vi "SendPPMSCommand_Rotator.vi"() -> ()   [LabVIEW 2016]
uses:
  Instance           1 31Saved   SendPPMSCommand_Rotator .vi
panel:
  out "Position while moving":dbl
  in  "Timeout":dbl
  in  "Delay":dbl=5.0
  out "error out":errorcluster
  in  "Slow down code\ndefault = 0":T1(ring)
  in  "Mode":u16(ring) items=["Move to position", "Move to limit", "Redefine current position", ""]
  in  "Position (deg)":dbl
  out "SendPPMSCommand Error 2":i32
  out "PpmsReply 2":string="0.000000"
  in  "PpmsCommand 2":string="$GETONE? 3"
  out "SendPPMSCommand Error":i32=1
  out "PpmsReply":string
  in  "Remote":bool
  in  "IP Address":string="127.0.0.0"
  # "Set Position"
  # "Final Position"
  # "Instrument Connection"
  # "Wait for Position"
  # "Note: normally one would use the GetPPMSItem VI to read the position on Channel 3. We use SendPPMSCmd here to show that we can read values this way."
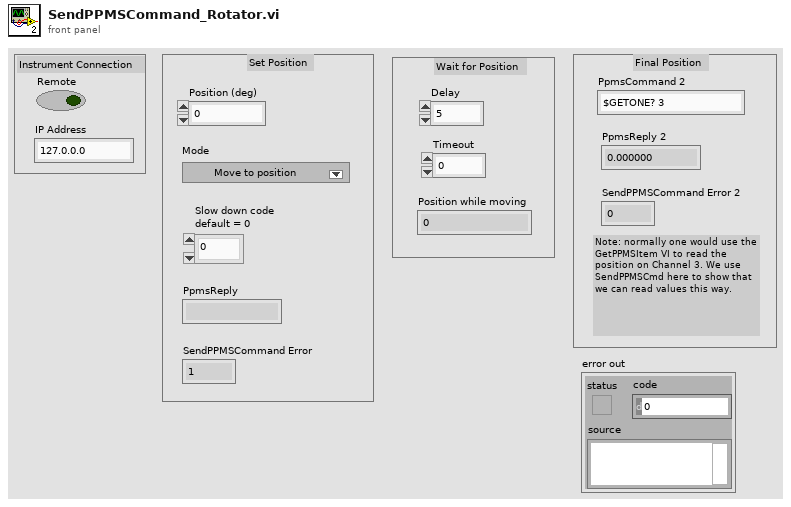
[diagram p1: front panel]
types:
  T1 = enum16{"0", "1", "2", "3", "4", "5", "6", "7", "8", "9", "10", "11", "12", "13", "14"}
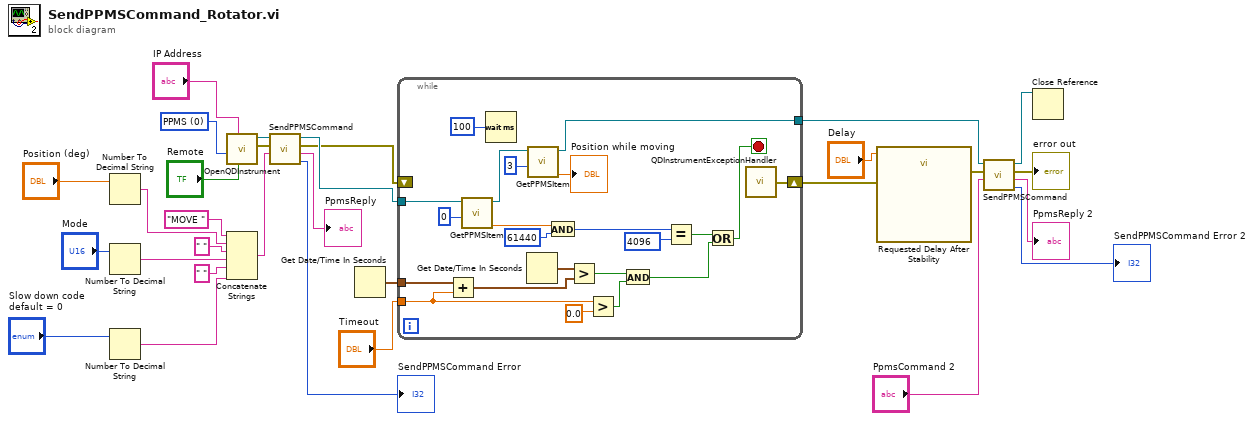
[diagram p0: block diagram]
diagram:
  w26 = 0 items=["PPMS", "VersaLab", "DynaCool", "SVSM"] ("Instrument Type")
  n1 = Number To Decimal String(number="Position (deg)") -> (decimal integer string=w18:string)  [unwired: 1 in]
  n2 = Number To Decimal String(number="Mode") -> (decimal integer string=w15:string)  [unwired: 1 in]
  n3 = Number To Decimal String(number="Slow down code\ndefault = 0") -> (decimal integer string=w12:string)  [unwired: 1 in]
  n4 = call "OpenQDInstrument.vi"("Remote"="Remote", "IP Address"="IP Address", "Instrument Type"=w26) -> ("error out"=w29:errorcluster, "Instrument Ref"=w30:refnum<k24>)  [unwired: 5 in]
  n5 = Concatenate Strings("MOVE " ("string"), w18, " " ("string"), w15, " " ("string"), w12) -> (w11:string)
  n6 = call "SendPPMSCommand.vi"("PpmsCommand"=w11, "error in (no error)"=w29, "Instrument Ref In"=w30) -> ("SendPPMSCommand Error"=→"SendPPMSCommand Error":i32, "PpmsReply"=→"PpmsReply":string, "error out"=w3:errorcluster, "Instrument Ref Out"=w6:refnum<k24>)  [unwired: 4 in, 1 out]
  n7 = Get Date/Time In Seconds() -> (seconds since 1Jan1904=w8:timestamp)
  n8 = while {
    shift-right: [w42] -> w10
    shift-left: w3 -> [_]
    tunnel: w8 -> [w51]
    tunnel: "Timeout" -> [w48]
    tunnel: w6 -> [w41]
    tunnel: [w32] -> w5
    stop <- w43 stop-if-true
    n9 = Add(x=w51, y=w48) -> (x+y=w49:timestamp)
    n10 = call "GetPPMSItem.vi"("Channel"=0, "Instrument Ref In"=w41) -> ("Result"=w35:dbl, "Instrument Ref Out"=w33:refnum<k24>)  [unwired: 2 in, 2 out]
    n11 = Wait (ms)(milliseconds to wait=u32 100) -> ()  [unwired: 1 out]
    n12 = Get Date/Time In Seconds() -> (seconds since 1Jan1904=w50:timestamp)
    n13 = call "GetPPMSItem.vi"("Channel"=3, "Instrument Ref In"=w33) -> ("Result"=→"Position while moving":dbl, "Instrument Ref Out"=w32:refnum<k24>)  [unwired: 2 in, 2 out]
    n14 = And(x=w35, y=61440) -> (x .and. y?=w39:i32)
    n15 = Greater?(x=w50, y=w49) -> (0:w46:bool)
    n16 = Greater?(x=w48, y=0.0) -> (0:w45:bool)
    n17 = And(x=w46, y=w45) -> (x .and. y?=w44:bool)
    n18 = Equal?(x=w39, y=4096) -> (x = y?=w37:bool)
    n19 = Or(x=w37, y=w44) -> (x .or. y?=w43:bool)
    n20 = call "QDInstrumentExceptionHandler.vi"() -> ("Error out"=w42:errorcluster)  [unwired: 1 in]
  }
  n21 = call "Requested Delay After Stability"("error in (no error)"=w10, "Delay Time (s)"="Delay") -> ("error out"=w2:errorcluster)  [unwired: 9 in]
  n22 = call "SendPPMSCommand.vi"("PpmsCommand"="PpmsCommand 2", "error in (no error)"=w2, "Instrument Ref In"=w5) -> ("SendPPMSCommand Error"=→"SendPPMSCommand Error 2":i32, "PpmsReply"=→"PpmsReply 2":string, "error out"=→"error out":errorcluster, "Instrument Ref Out"=w4:refnum<k24>)  [unwired: 4 in, 1 out]
  n23 = Close Reference(reference=w4) -> ()  [unwired: 1 in, 1 out]
